vi "Create Batch Response.vi"(8 "error in (no error)":errorcluster, 10 "results":variant[](array[variant]), 11 "JSON-RPC in":refnum<class "JSON-RPC.lvclass">) -> (0 "error out":errorcluster, 2 "Response":string, 3 "JSON-RPC out":refnum<class "JSON-RPC.lvclass">)   [LabVIEW 2019, in "JSON-RPC.lvclass"]
uses:
  JSON-RPC.lvclass
  JSON-RPC.lvclass/JSON-RPC.ctl
  Response/Response.lvclass
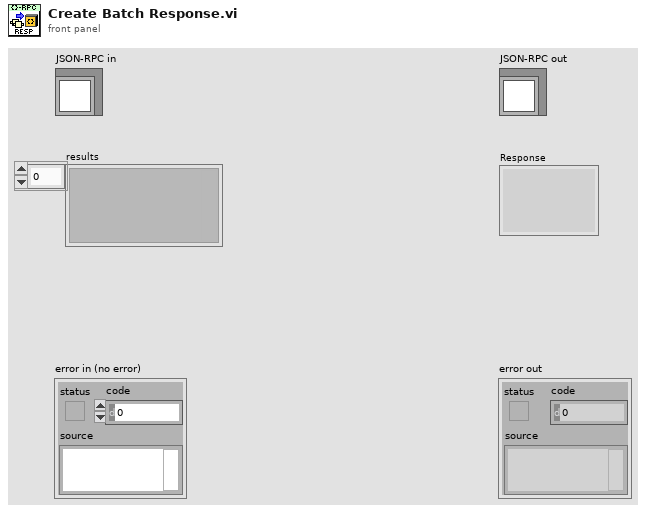
[diagram p1: front panel]
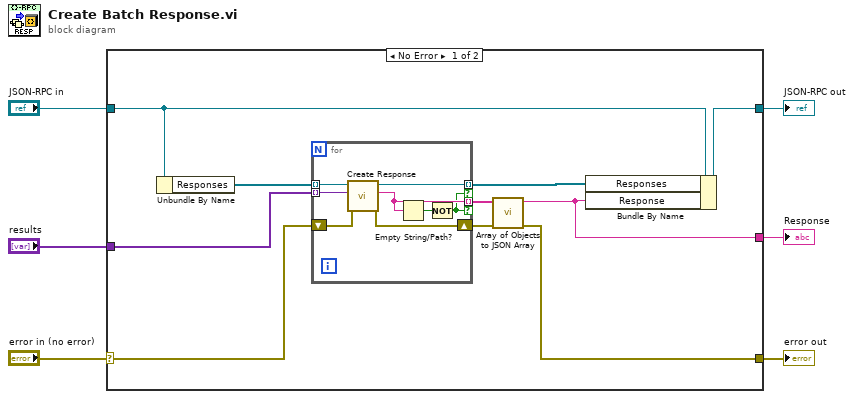
[diagram p0: block diagram]
diagram:
  n1 = case shown="No Error" "error in (no error)" {
    selector: "error in (no error)" -> [w11 w26]
    tunnel: [w7 w26] -> w5
    tunnel: [w15 w25] -> w4
    tunnel: "results" -> [w12 _]
    tunnel: [w9 _] -> w2
    tunnel: "JSON-RPC in" -> [w14 w25]
    frame No Error {
      n2 = Unbundle By Name(w14) -> ("Responses"=w13:refnum<class "Response.lvclass">[])
      n3 = for {
        tunnel: [w24] -> w16 mode=indexing if=w17
        tunnel: [w18] -> w10 mode=indexing if=w17
        tunnel: w13 -> [w22] mode=indexing
        tunnel: w12 -> [w21] mode=indexing
        shift-right: [w23] -> w8
        shift-left: w11 -> [w20]
        n4 = call "Create Response.vi"("error in (no error)"=w20, "result"=w21, "Response"=w22) -> ("error out"=w23:errorcluster, "JSON Response"=w18:string, "Response out"=w24:refnum<class "Response.lvclass">)  [unwired: 6 in]
        n5 = Empty String/Path?(string/path=w18) -> (empty?=w19:bool)
        n6 = Not(x=w19) -> (.not. x?=w17:bool)
      }
      n7 = call "Array of Objects to JSON Array.vi"("error in (no error)"=w8, "Array of JSON"=w10) -> ("error out"=w7:errorcluster, "JSON Array"=w9:string)  [unwired: 8 in]
      n8 = Bundle By Name(cluster=w14, "Responses"=w16, "Response"=w9) -> (w15:refnum<class "JSON-RPC.lvclass">)
    }
    frame Error {
    }
  }
  "error out" <- w5
  "JSON-RPC out" <- w4
  "Response" <- w2
